vi "UI-电源头正面标签凹凸检测.vi"(8 "error in (no error)":errorcluster caption="错误输入（无错误）", 11 "名称或相对路径":string="Template Program") -> (0 "error in (no error) 2":errorcluster caption="错误输入（无错误）")   [LabVIEW 2017]
uses:
  Picture/SaveButtom.ctl
  Global System.vi
  <vilib>/Utility/xml.llb/Write to XML File(string).vi
panel:
  in  "获取图像":bool
  in  "创建模板":bool
  in  "保存图像":bool
  out "添加的路径":path
  in  "刷新":bool
  in  "测试按钮":bool
  in  "保存按钮":bool
  in  "Main":enum32{"主参数", "颜色模板匹配参数 ", "测试效果"}(tab)
  in  "UI电源线正面凹凸基础参数":T1={"IsNorImage"=TRUE, "Exposure Values"=100289, "ImagePath"=path "C:/Users/hedongpo/Desktop/514-hdp/Alignment Assemble System/Test Picture/B/3.bmp"} caption="参数界面" {"Exposure Values" scale=0.0..200000.0}
  in  "UI电源线正面凹凸参数":T2={"Min Radius"=7.0, "Max Radius"=11.0, "Max Number"=11.0}
  out "结果":bool
  out "原始图像":T3(plugin-control)
  out "大小":i32
  out "路径输出":path
  in  "Vision Paramter Save Buttom":T4
  out "system time":string
  in  "取消按钮":bool
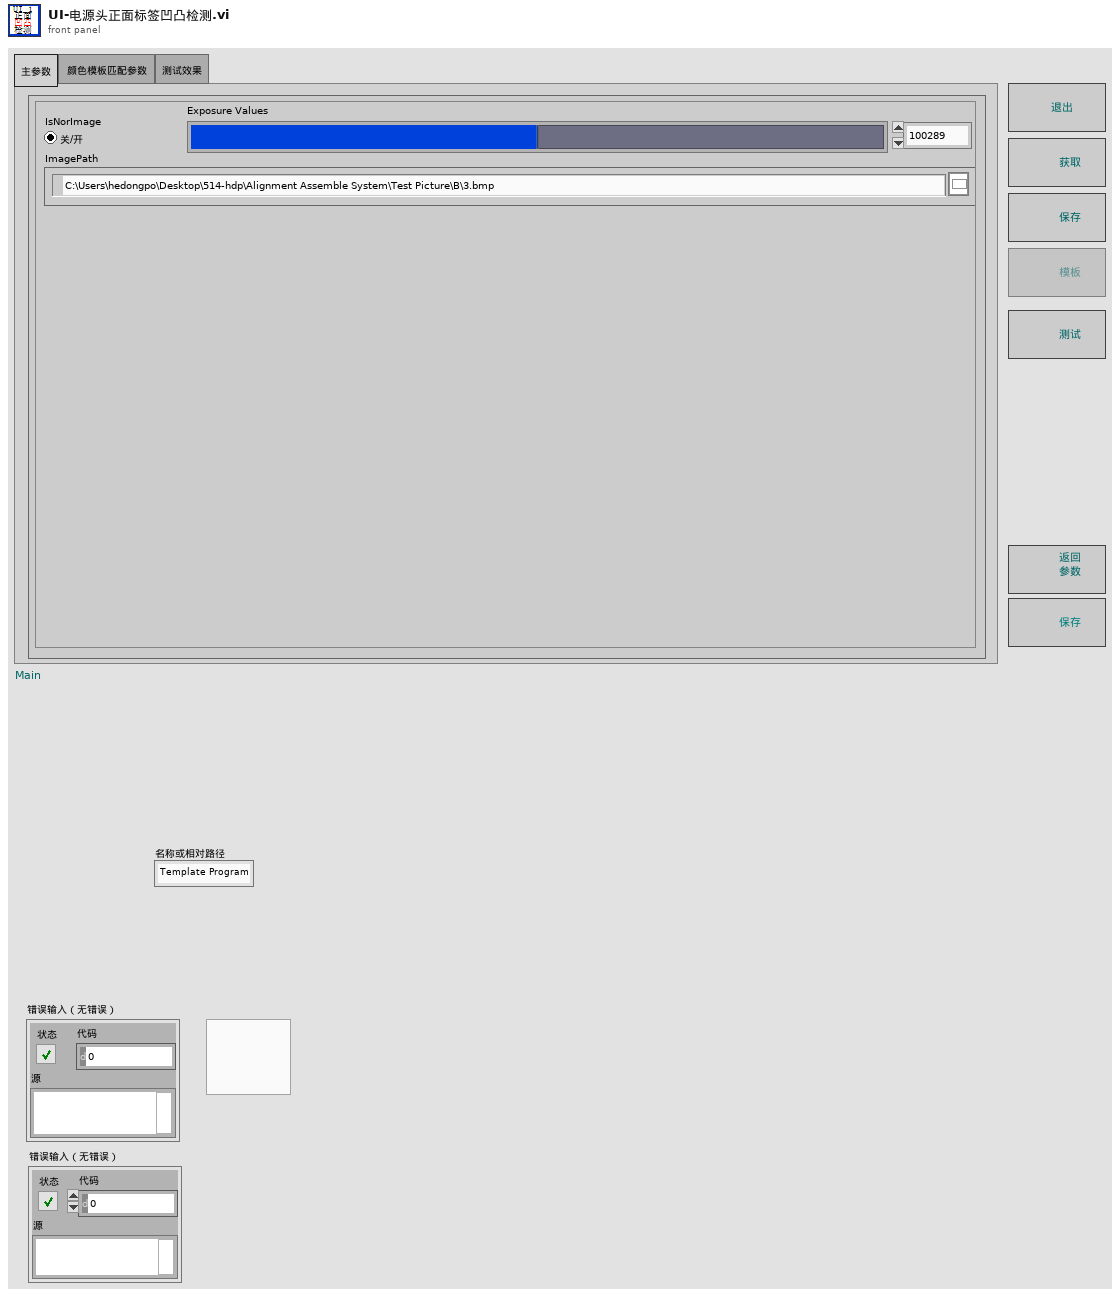
[diagram p1: front panel]
types:
  T1 = cluster{"IsNorImage":bool, "Exposure Values":u32, "ImagePath":path}
  T2 = cluster{"Min Radius":sgl, "Max Radius":sgl, "Max Number":sgl}
  T3 = typedef "IMAQ Image.ctl" = refnum<image>
  T4 = typedef "SaveButtom.ctl" = bool
  T5 = cluster{"index":i32, "this vi":refnum<vi>, "error out":errorcluster}
  T6 = cluster{"master data":string, "priority":u16, "secondary data":string[]}
  T7 = cluster{"case name":string[], "queue array":refnum<queue>[]}
  T8 = cluster{"Pos. X":i32, "Pos. Y":i32, "Radius":i32, "Core Area":i32}[]
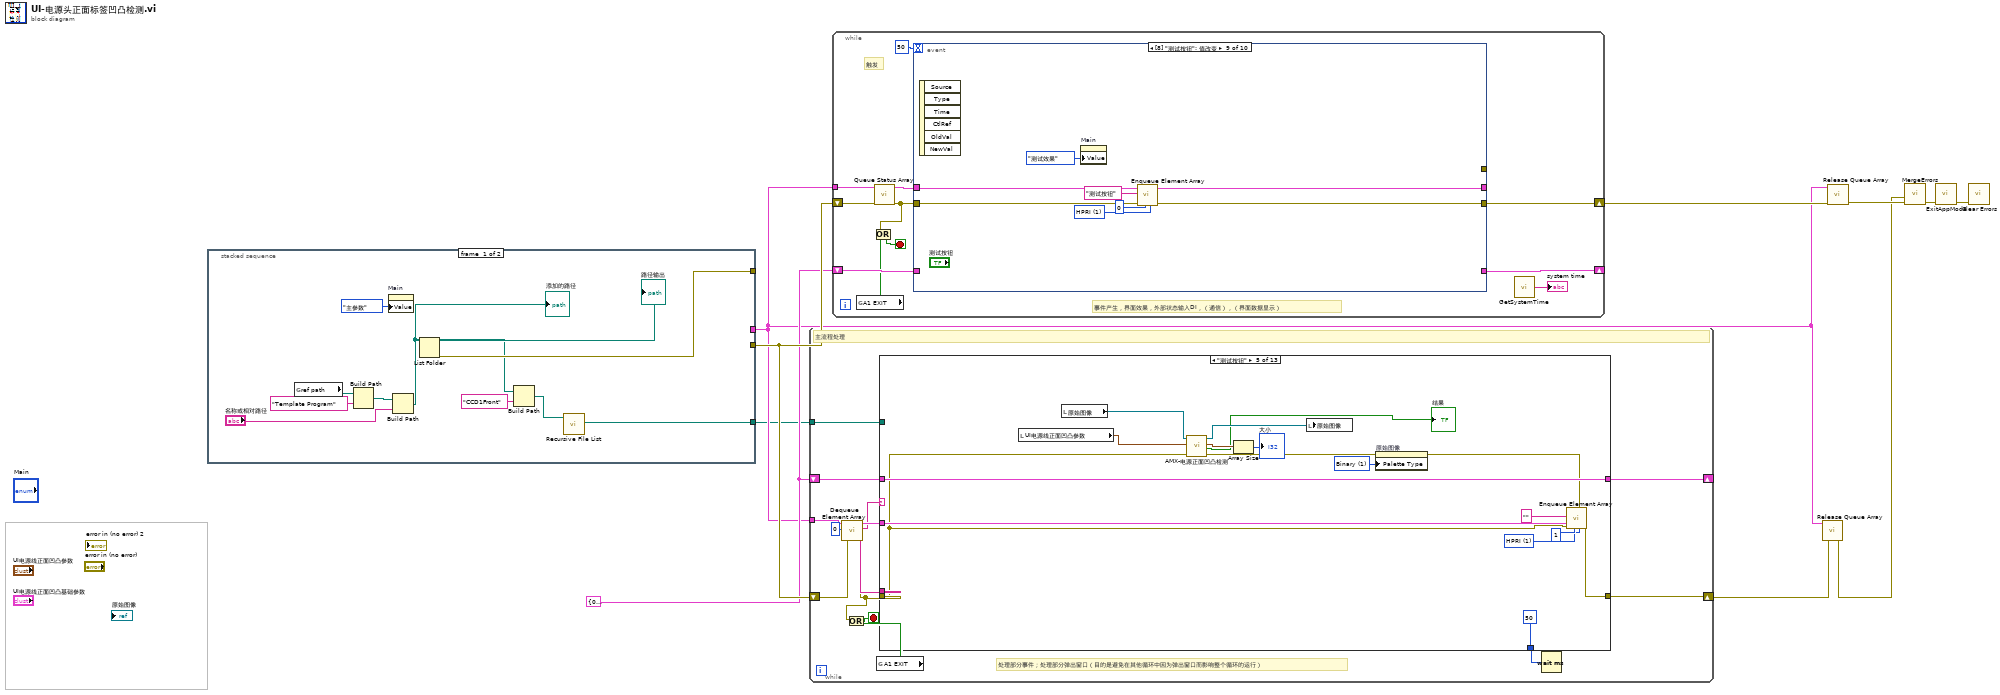
[diagram p0: block diagram]
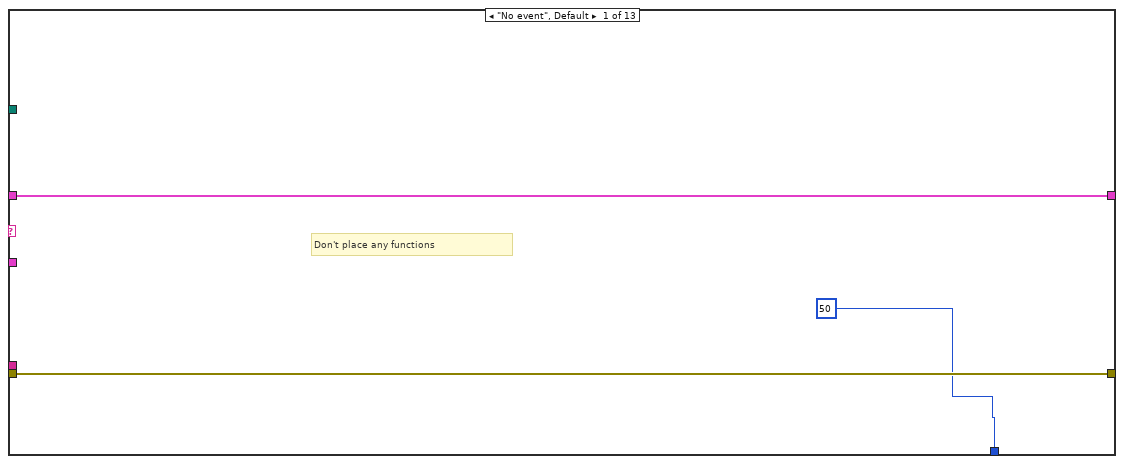
[diagram p2: hidden frame]
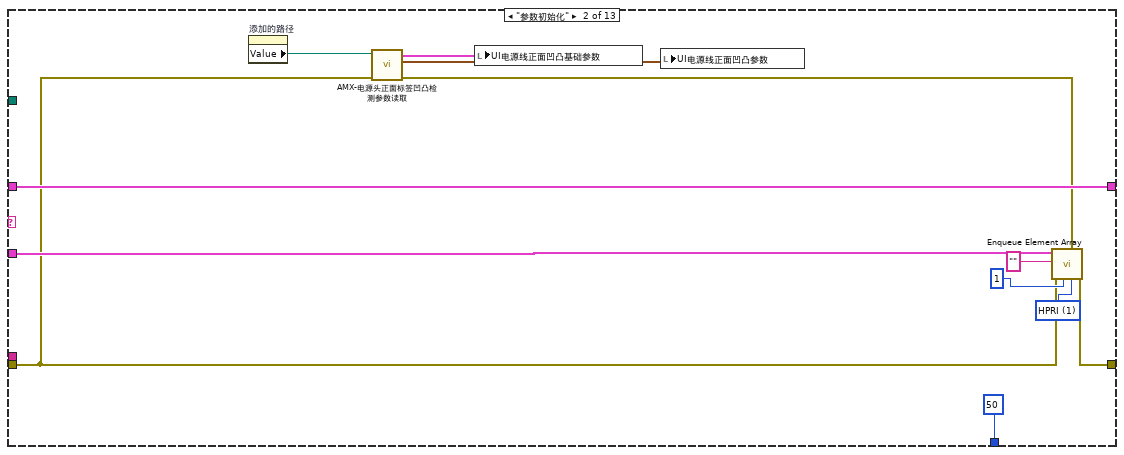
[diagram p3: hidden frame]
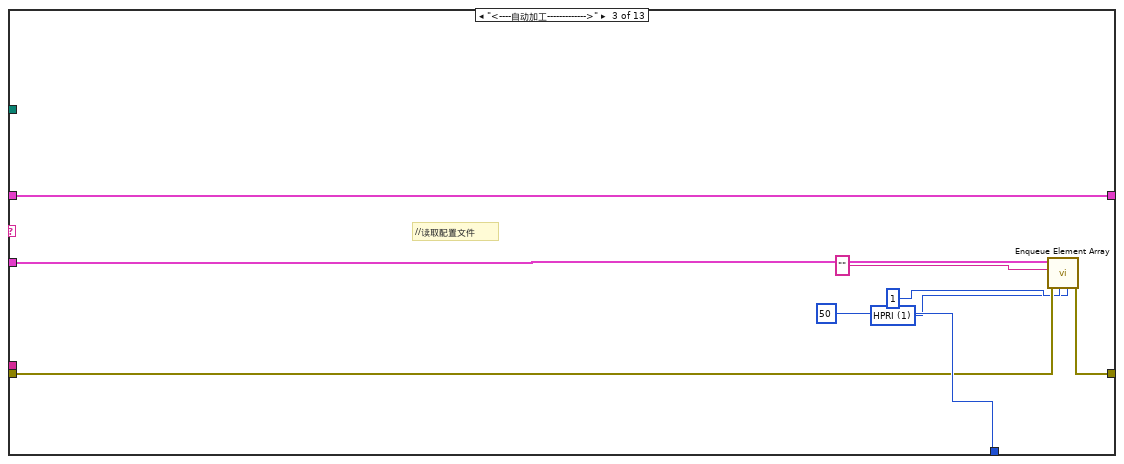
[diagram p4: hidden frame]
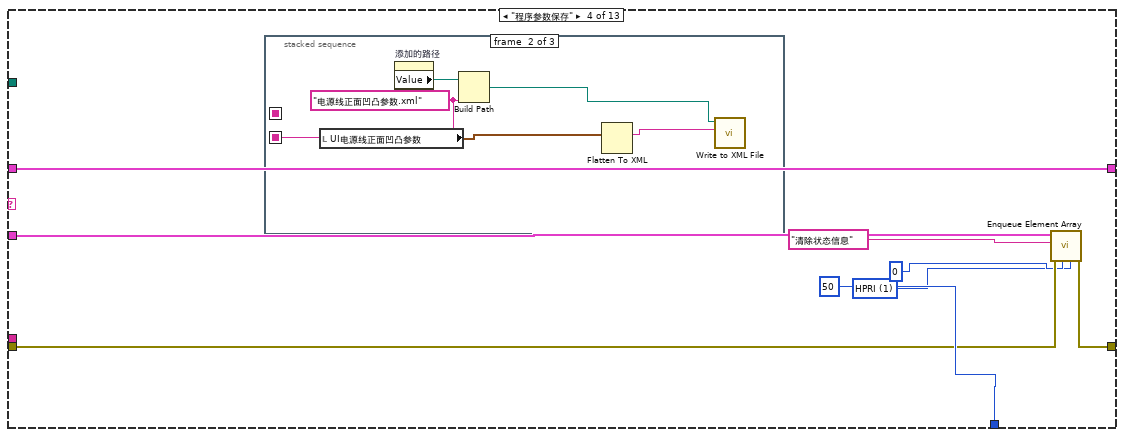
[diagram p5: hidden frame]
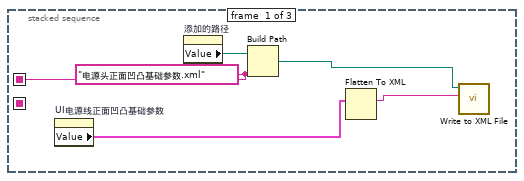
[diagram p6: hidden frame]
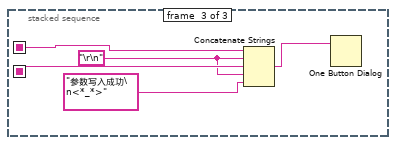
[diagram p7: hidden frame]
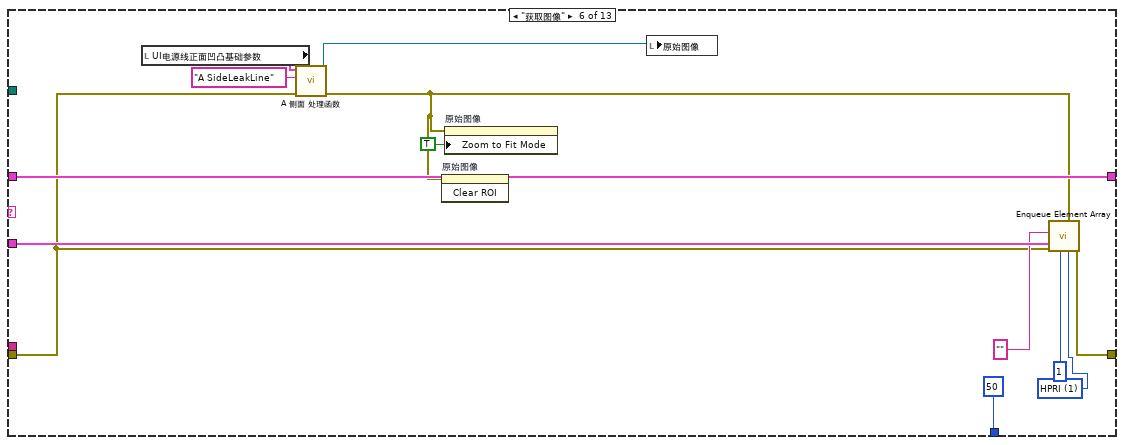
[diagram p8: hidden frame]
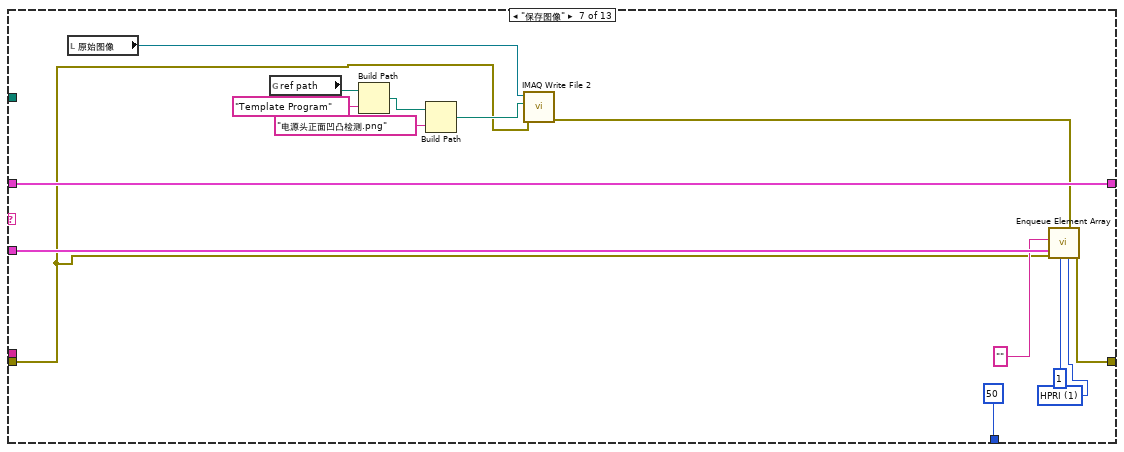
[diagram p9: hidden frame]
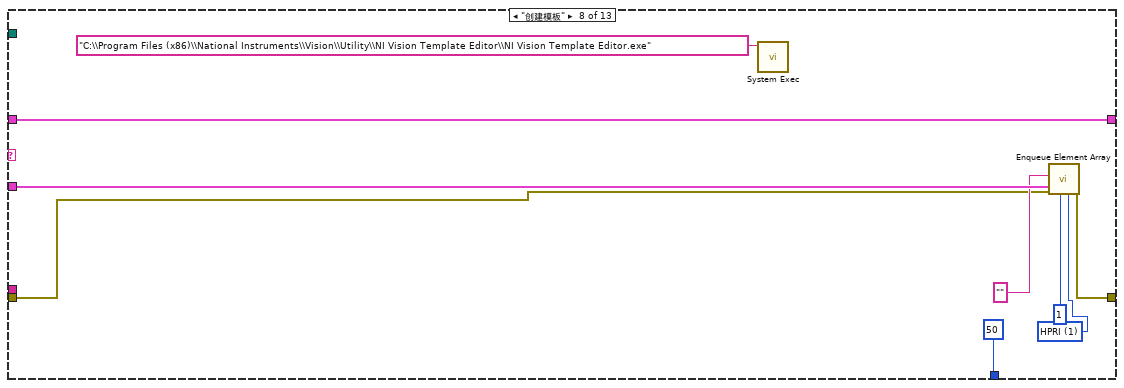
[diagram p10: hidden frame]
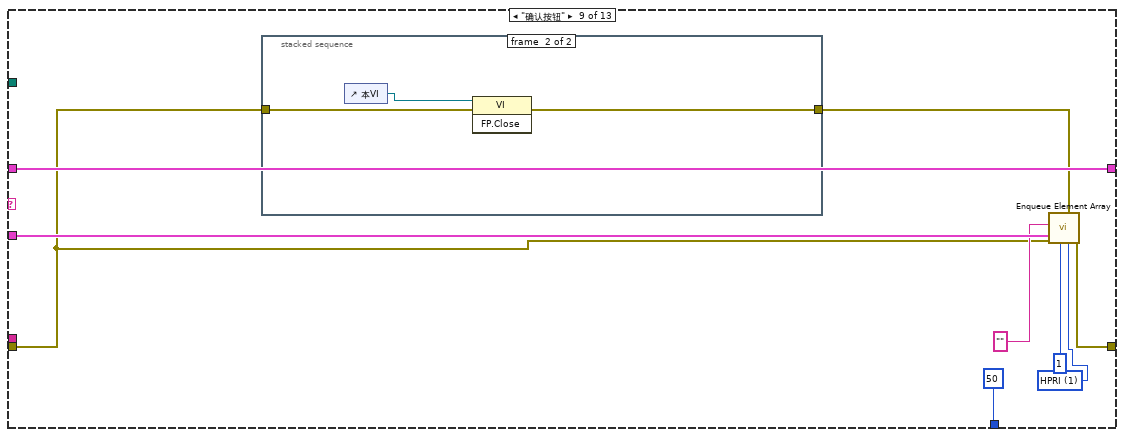
[diagram p11: hidden frame]
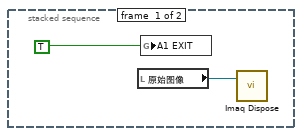
[diagram p12: hidden frame]
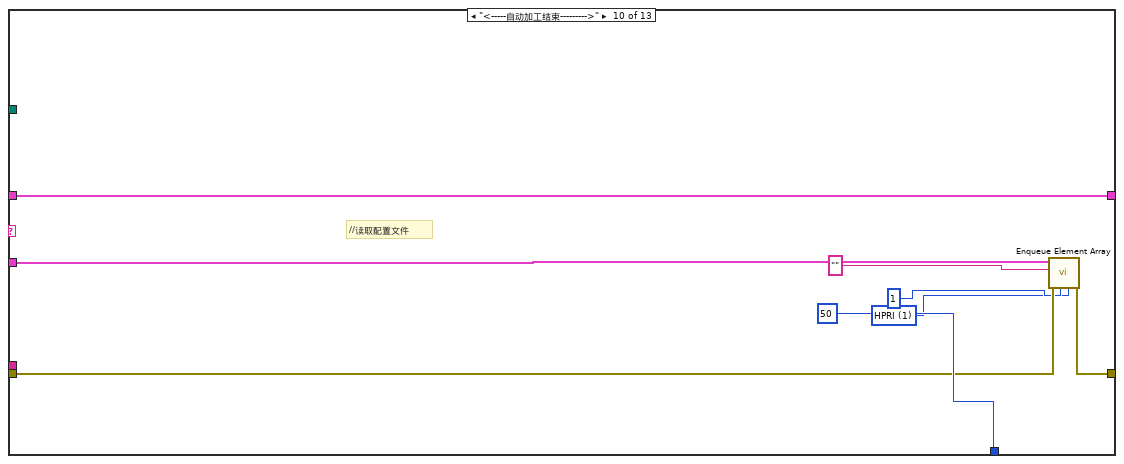
[diagram p13: hidden frame]
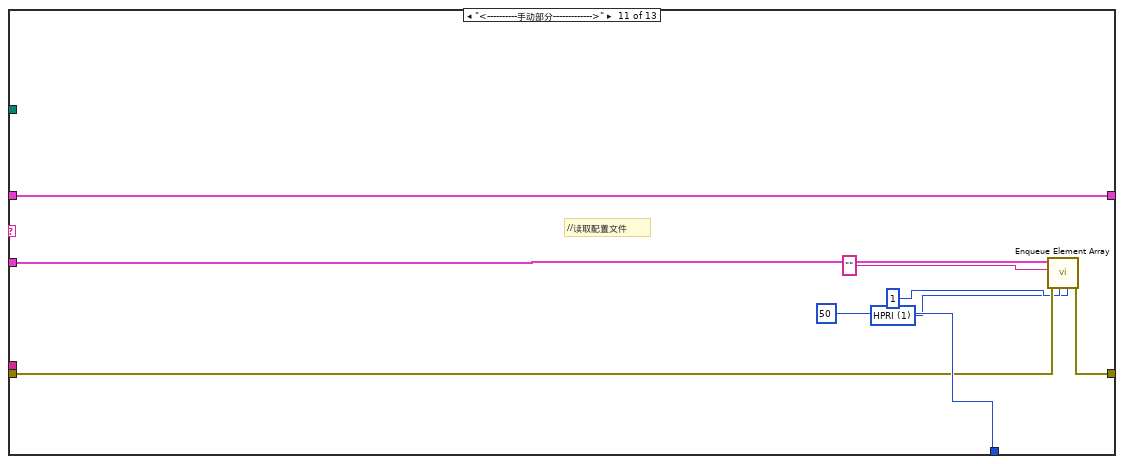
[diagram p14: hidden frame]
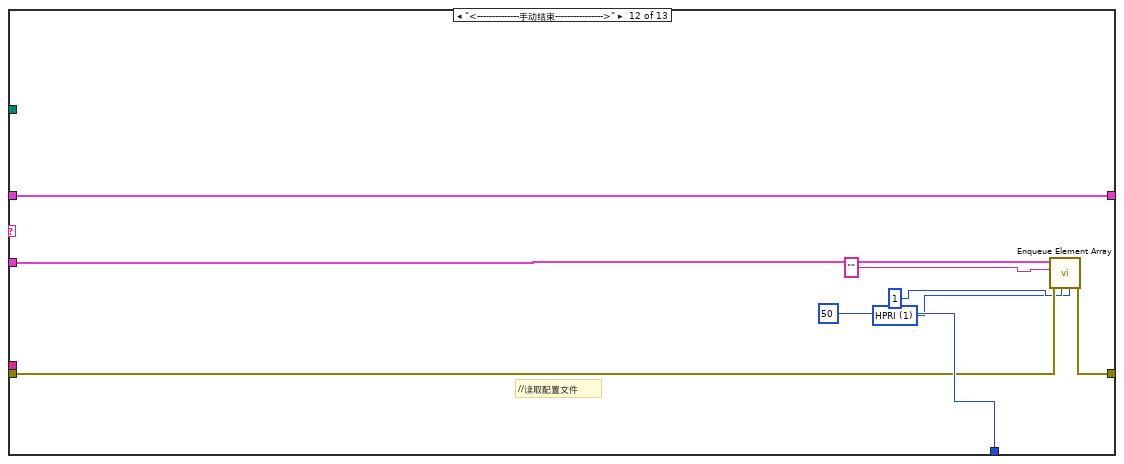
[diagram p15: hidden frame]
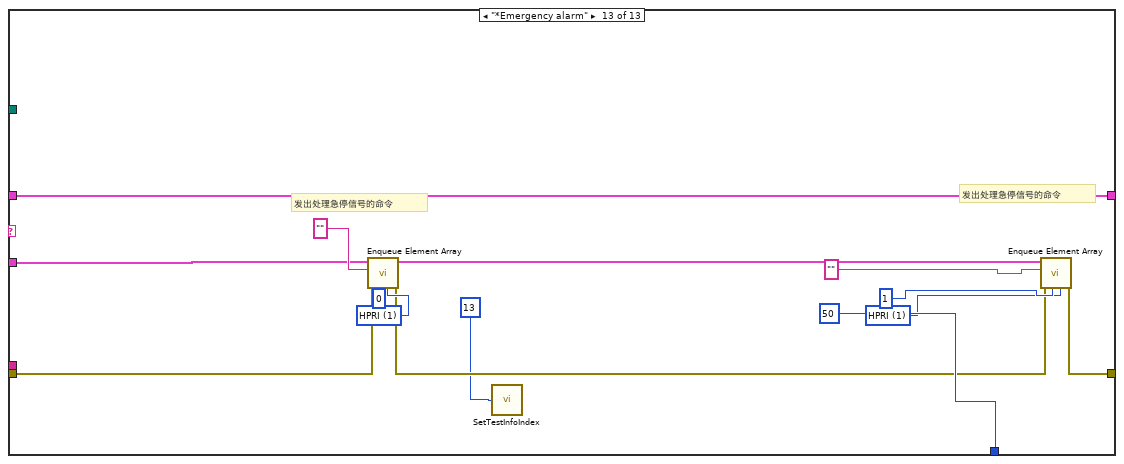
[diagram p16: hidden frame]
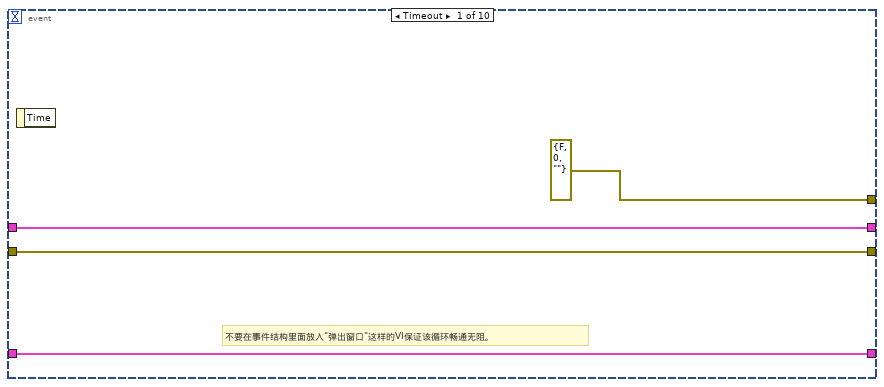
[diagram p17: hidden frame]
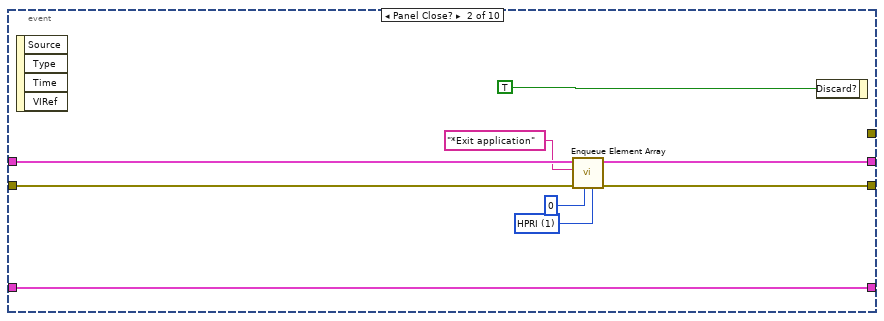
[diagram p18: hidden frame]
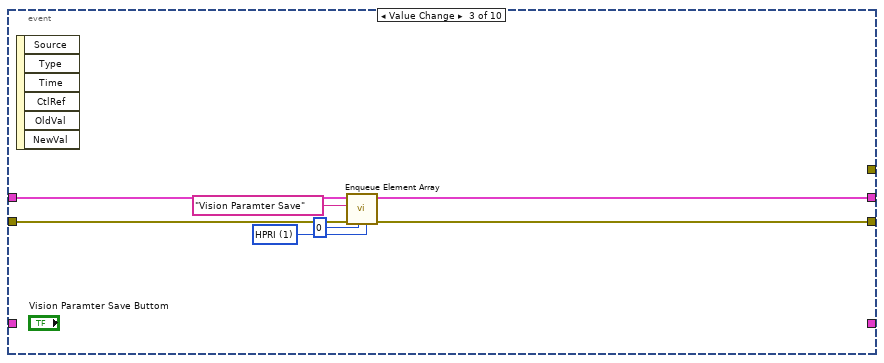
[diagram p19: hidden frame]
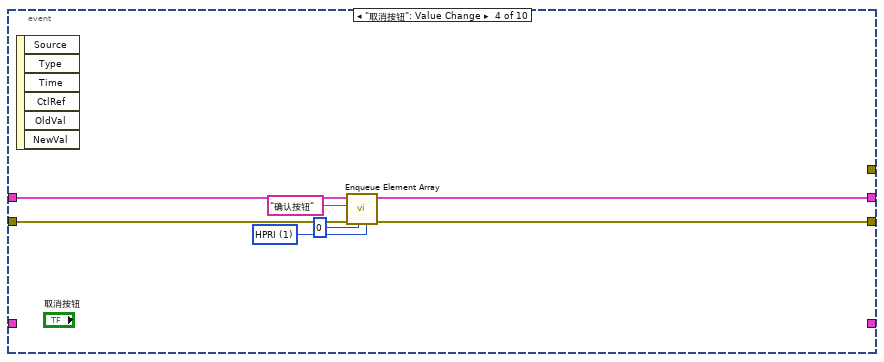
[diagram p20: hidden frame]
diagram:
  w5 = T5 {"index"=0, "this vi"=refnum, "error out"={"status"=FALSE, "code"=0, "source"=""}} ("parameter buffer")
  n1 = stacked-sequence {
    tunnel: [w20 _] -> _
    tunnel: [_ w23] -> w6
    tunnel: [_ w22] -> w2
    tunnel: [w11 _] -> w1
    frame #0 {
      n2 = global read "Global System.vi" "ref path"() -> (w18:path)
      n3 = Build Path(base path=w18, name or relative path="Template Program" ("名称或相对路径")) -> (appended path=w16:path)
      n4 = property on="Main" class="TabCtl (严格)"("Value"=enum32{"主参数", "颜色模板匹配参数 ", "测试效果"}."主参数" ("Main")) -> ()  [unwired: 2 in, 2 out]
      n5 = Build Path(base path=w16, name or relative path="名称或相对路径") -> (appended path=w12:path)
      "添加的路径" <- w12
      n6 = List Folder(path=w12) -> (path out=→"路径输出":path, error out=w20:errorcluster)  [unwired: 3 in, 2 out]
      n7 = Build Path(base path=w12, name or relative path="CCD1Front" ("名称或相对路径")) -> (appended path=w13:path)
      n8 = call <vilib>:"Recursive File List.vi"("Folder Path"=w13) -> ("All Files in Dir"=w11:path[])  [unwired: 6 in, 4 out]
    }
    frame #1 {
      w31 = string[] ["comm queue1", "data queue 11", "data queue 12", "data queue 13", "data queue 14"]  # queue name
      w32 = 4  # queue num
      w33 = T6 {"master data"="", "priority"=0, "secondary data"=[]}  # element data type
      n9 = call "Obtain Queue Array.vi"("queue name"=w31, "element data type"=w33, "queue num"=w32) -> ("error out"=w27:errorcluster, "queue out"=w28:T7)  [unwired: 2 in, 1 out]
      n10 = call "Enqueue Element Array.vi"("queue index"=0, "error in"=w27, "master data"="参数初始化", "queue in"=w28) -> ("error out"=w26:errorcluster, "queue out"=w25:T7)  [unwired: 6 in]
      n11 = disable-structure shown="启用" {
        disable-tunnel: w26 -> [w39 w40]
        disable-tunnel: w25 -> [w38 w41]
        disable-tunnel: "Loading Variable" ("master data") -> [w37 _]
        disable-tunnel: [w35 w40] -> w23
        disable-tunnel: [w34 w41] -> w22
        frame Disabled {
          n12 = call "Enqueue Element Array.vi"("queue index"=12, "error in"=w39, "master data"=w37, "queue in"=w38) -> ("error out"=w35:errorcluster, "queue out"=w34:T7)  [unwired: 6 in]
        }
        frame Enabled {
        }
      }
    }
  }
  n13 = while {
    shift-right: [w55] -> w4
    shift-left: w6 -> [w46]
    shift-right: [w52] -> _
    shift-left: w5 -> [w53]
    tunnel: w2 -> [w48]
    tunnel: w1 -> [w42]
    stop <- w43 stop-if-true
    # "处理部分事件；处理部分弹出窗口（目的是避免在其他循环中因为弹出窗口而影响整个循环的运行）"
    # "主流程处理"
    n14 = call "Dequeue Element Array.vi"("queue in"=w48, "queue index"=0, "error in"=w46) -> ("queue out"=w51:T7, "master data"=w50:string, "secondary data"=w49:string[], "error out"=w45:errorcluster)  [unwired: 2 in, 1 out]
    n15 = global read "Global System.vi" "A1 EXIT"() -> (w44:bool)
    n16 = Or(x=w45, y=w44) -> (x .or. y?=w43:bool)
    n17 = case shown="\"测试按钮\"" w50 {
      tunnel: w51 -> [_ w69 w77 w79 w117 w130 w145 w154 w163 w176 w184 w192 w198]
      tunnel: w45 -> [w57 w63 w73 w83 w109 w121 w132 w148 w157 w172 w180 w188 w195]
      tunnel: [w57 w68 w76 w85 w116 w129 w144 w153 w162 w175 w183 w191 w206] -> w55
      tunnel: [50 50 50 50 50 50 50 50 50 50 50 50 50] -> w54
      tunnel: w53 -> [w58 w64 w74 w80 w112 w125 w140 w149 w158 w173 w181 w189 w204]
      tunnel: [w58 w64 w74 w80 w112 w125 w140 w149 w158 w173 w181 w189 w204] -> w52
      tunnel: w49 -> [_ _ _ _ _ _ _ _ _ _ _ _ _]
      tunnel: w42 -> [_ _ _ _ _ _ _ _ _ _ _ _ _]
      frame "No event", Default {
        # "Don't place any functions"
      }
      frame "参数初始化" {
        w65 = u16 1 items=["HPRI"=1, "LPRI"=0] ("priority")
        n18 = property on="添加的路径" class="Path"() -> ("Value"=w61:path)  [unwired: 2 in, 2 out]
        n19 = call "AMX-电源头正面标签凹凸检测参数读取.vi"("error in (no error)"=w63, "基路径"=w61) -> ("error out"=w62:errorcluster, "UI电源线正面凹凸参数"=w59:T2, "UI电源线正面漏线基础参数"=w60:T1)  [unwired: 6 in]
        n20 = local write "UI电源线正面凹凸基础参数"(w60) -> ()
        n21 = local write "UI电源线正面凹凸参数"(w59) -> ()
        n22 = call "Enqueue Element Array.vi"("priority"=w65, "device error in"=w62, "queue index"=1, "error in"=w63, "master data"="" ("Element 1"), "queue in"=w69) -> ("error out"=w68:errorcluster)  [unwired: 4 in, 1 out]
      }
      frame "<----自动加工------------->" {
        w71 = u16 1 items=["HPRI"=1, "LPRI"=0] ("priority")
        # "//读取配置文件"
        n23 = call "Enqueue Element Array.vi"("priority"=w71, "queue index"=1, "error in"=w73, "master data"="" ("Element 1"), "queue in"=w77) -> ("error out"=w76:errorcluster)  [unwired: 5 in, 1 out]
      }
      frame "程序参数保存" {
        w81 = u16 1 items=["HPRI"=1, "LPRI"=0] ("priority")
        n24 = stacked-sequence {
          seq-local: [w87 _ _] -> [_ _ w100]
          seq-local: [_ w93 _] -> [_ _ w98]
          frame #0 {
            w87 = "电源头正面凹凸基础参数.xml" ("名称或相对路径")
            n25 = property on="UI电源线正面凹凸基础参数" class="Clust (严格)"() -> ("Value"=w90:T1)  [unwired: 2 in, 2 out]
            n26 = property on="添加的路径" class="Path"() -> ("Value"=w91:path)  [unwired: 2 in, 2 out]
            n27 = Build Path(base path=w91, name or relative path=w87) -> (appended path=w88:path)
            n28 = Flatten To XML(anything=w90) -> (xml string=w89:string)
            n29 = call-poly <vilib>:"Write to XML File.vi"("XML Input"=w89, "XML File Path"=w88) -> ()  [unwired: 7 in, 3 out]
          }
          frame #1 {
            w93 = "电源线正面凹凸参数.xml" ("名称或相对路径")
            n30 = local read "UI电源线正面凹凸参数"() -> (w92:T2)
            n31 = property on="添加的路径" class="Path"() -> ("Value"=w96:path)  [unwired: 2 in, 2 out]
            n32 = Build Path(base path=w96, name or relative path=w93) -> (appended path=w94:path)
            n33 = Flatten To XML(anything=w92) -> (xml string=w95:string)
            n34 = call-poly <vilib>:"Write to XML File.vi"("XML Input"=w95, "XML File Path"=w94) -> ()  [unwired: 7 in, 3 out]
          }
          frame #2 {
            w97 = "\r\n"
            n35 = Concatenate Strings(w100, w97, w98, w97, "参数写入成功\n<*_*>" ("消息")) -> (w99:string)
            n36 = One Button Dialog(message=w99) -> ()  [unwired: 1 in, 1 out]
          }
        }
        n37 = call "Enqueue Element Array.vi"("priority"=w81, "queue index"=0, "error in"=w83, "master data"="清除状态信息" ("Element 1"), "queue in"=w79) -> ("error out"=w85:errorcluster)  [unwired: 5 in, 1 out]
      }
      frame "测试按钮" {
        w104 = u32 1 items=["Grayscale", "Binary", "Gradient", "Rainbow", "Temperature", "User Defined", "Binary 16 Bit", "Gradient 16 Bit", "Rainbow 16 Bit", "Temperature 16 Bit", "User Defined 16 Bit"] ("Palette:Palette Type")
        w113 = u16 1 items=["HPRI"=1, "LPRI"=0] ("priority")
        n38 = local read "UI电源线正面凹凸参数"() -> (w103:T2)
        n39 = local read "原始图像"() -> (w111:T3)
        n40 = call "AMX-电源正面凹凸检测.vi"("error in (no error)"=w109, "UI电源线正面漏线参数"=w103, "Image in"=w111) -> ("error out"=w106:errorcluster, "x >= y?"=→"结果":bool, "Circles Data (calibrated) (Circle Detection 1)"=w108:T8, "Image out"=w110:T3)  [unwired: 5 in]
        n41 = Array Size(array=w108) -> (size(s)=→"大小":i32)
        n42 = local write "原始图像"(w110) -> ()
        n43 = property on="原始图像" class="ImageControl"(error in=w106, "Palette Type"=w104) -> (error out=w105:errorcluster)  [unwired: 1 in, 1 out]
        n44 = call "Enqueue Element Array.vi"("priority"=w113, "device error in"=w105, "queue index"=1, "error in"=w109, "master data"="" ("Element 1"), "queue in"=w117) -> ("error out"=w116:errorcluster)  [unwired: 4 in, 1 out]
      }
      frame "获取图像" {
        w126 = u16 1 items=["HPRI"=1, "LPRI"=0] ("priority")
        n45 = local read "UI电源线正面凹凸基础参数"() -> (w123:T1)
        n46 = call "A 侧面 处理函数.vi"("error in (no error)"=w121, "Image Name"="A SideLeakLine", "ParamsUI"=w123) -> ("error out"=w119:errorcluster, "Image out"=w122:T3)  [unwired: 5 in, 2 out]
        n47 = invoke on="原始图像" class="ImageControl" method="Clear ROI"(error in=w119) -> ()  [unwired: 2 in, 3 out]
        n48 = property on="原始图像" class="ImageControl"(error in=w119, "Zoom to Fit Mode"=TRUE) -> ()  [unwired: 1 in, 2 out]
        n49 = local write "原始图像"(w122) -> ()
        n50 = call "Enqueue Element Array.vi"("priority"=w126, "device error in"=w119, "queue index"=1, "error in"=w121, "master data"="" ("Element 1"), "queue in"=w130) -> ("error out"=w129:errorcluster)  [unwired: 4 in, 1 out]
      }
      frame "保存图像" {
        w141 = u16 1 items=["HPRI"=1, "LPRI"=0] ("priority")
        n51 = local read "原始图像"() -> (w133:T3)
        n52 = global read "Global System.vi" "ref path"() -> (w139:path)
        n53 = Build Path(base path=w139, name or relative path="Template Program" ("名称或相对路径")) -> (appended path=w137:path)
        n54 = Build Path(base path=w137, name or relative path="电源头正面凹凸检测.png" ("名称或相对路径")) -> (appended path=w135:path)
        n55 = call-poly "IMAQ Write File 2"("error in (no error)"=w132, "File Path"=w135, "Image"=w133) -> ("error out"=w134:errorcluster)  [unwired: 7 in, 1 out]
        n56 = call "Enqueue Element Array.vi"("priority"=w141, "device error in"=w134, "queue index"=1, "error in"=w132, "master data"="" ("Element 1"), "queue in"=w145) -> ("error out"=w144:errorcluster)  [unwired: 4 in, 1 out]
      }
      frame "创建模板" {
        w150 = u16 1 items=["HPRI"=1, "LPRI"=0] ("priority")
        n57 = call <vilib>:"System Exec.vi"("command line"="C:\\Program Files (x86)\\National Instruments\\Vision\\Utility\\NI Vision Template Editor\\NI Vision Template Editor.exe") -> ()  [unwired: 7 in, 4 out]
        n58 = call "Enqueue Element Array.vi"("priority"=w150, "queue index"=1, "error in"=w148, "master data"="" ("Element 1"), "queue in"=w154) -> ("error out"=w153:errorcluster)  [unwired: 5 in, 1 out]
      }
      frame "确认按钮" {
        w159 = u16 1 items=["HPRI"=1, "LPRI"=0] ("priority")
        n59 = stacked-sequence {
          tunnel: w157 -> [_ w168]
          tunnel: [_ w167] -> w156
          frame #0 {
            n60 = local read "原始图像"() -> (w165:T3)
            n61 = global write "Global System.vi" "A1 EXIT"(TRUE ("EXIT")) -> ()
            n62 = call "Imaq Dispose"("Image"=w165) -> ()  [unwired: 5 in, 1 out]
          }
          frame #1 {
            n63 = control-ref of="本VI"() -> (w169:refnum<vi>)
            n64 = invoke class="VI" method="FP.Close"(reference=w169, error in=w168) -> (error out=w167:errorcluster)  [unwired: 1 in, 2 out]
          }
        }
        n65 = call "Enqueue Element Array.vi"("priority"=w159, "device error in"=w156, "queue index"=1, "error in"=w157, "master data"="" ("Element 1"), "queue in"=w163) -> ("error out"=w162:errorcluster)  [unwired: 4 in, 1 out]
      }
      frame "<-----自动加工结束--------->" {
        w170 = u16 1 items=["HPRI"=1, "LPRI"=0] ("priority")
        # "//读取配置文件"
        n66 = call "Enqueue Element Array.vi"("priority"=w170, "queue index"=1, "error in"=w172, "master data"="" ("Element 1"), "queue in"=w176) -> ("error out"=w175:errorcluster)  [unwired: 5 in, 1 out]
      }
      frame "<----------手动部分------------->" {
        w178 = u16 1 items=["HPRI"=1, "LPRI"=0] ("priority")
        # "//读取配置文件"
        n67 = call "Enqueue Element Array.vi"("priority"=w178, "queue index"=1, "error in"=w180, "master data"="" ("Element 1"), "queue in"=w184) -> ("error out"=w183:errorcluster)  [unwired: 5 in, 1 out]
      }
      frame "<--------------手动结束---------------->" {
        w186 = u16 1 items=["HPRI"=1, "LPRI"=0] ("priority")
        # "//读取配置文件"
        n68 = call "Enqueue Element Array.vi"("priority"=w186, "queue index"=1, "error in"=w188, "master data"="" ("Element 1"), "queue in"=w192) -> ("error out"=w191:errorcluster)  [unwired: 5 in, 1 out]
      }
      frame "*Emergency alarm" {
        w201 = u16 1 items=["HPRI"=1, "LPRI"=0] ("priority")
        w202 = u16 1 items=["HPRI"=1, "LPRI"=0] ("priority")
        # "发出处理急停信号的命令"
        # "发出处理急停信号的命令"
        n69 = call "Enqueue Element Array.vi"("priority"=w201, "queue index"=0, "error in"=w195, "master data"="" ("Element 1"), "queue in"=w198) -> ("error out"=w196:errorcluster, "queue out"=w197:T7)  [unwired: 5 in]
        n70 = call "SetTestInfoIndex.vi"("test info index"=13) -> ()
        n71 = call "Enqueue Element Array.vi"("priority"=w202, "queue index"=1, "error in"=w196, "master data"="" ("Element 1"), "queue in"=w197) -> ("error out"=w206:errorcluster)  [unwired: 5 in, 1 out]
      }
    }
    n72 = Wait (ms)(milliseconds to wait=w54) -> ()  [unwired: 1 out]
  }
  n73 = while {
    shift-right: [w211] -> w7
    shift-left: w6 -> [w215]
    shift-right: [w213] -> _
    shift-left: w5 -> [w214]
    tunnel: w2 -> [w217]
    stop <- w208 stop-if-true
    # "触发"
    # "事件产生，界面效果，外部状态输入DI，（通信），（界面数据显示）"
    n74 = global read "Global System.vi" "A1 EXIT"() -> (w209:bool)
    n75 = call "Queue Status Array.vi"("error in (no error)"=w215, "queue in"=w217) -> ("error out"=w210:errorcluster, "queue out"=w212:T7)  [unwired: 4 in]
    n76 = Or(x=w210, y=w209) -> (x .or. y?=w208:bool)
    n77 = event shown="[8] \"测试按钮\": 值改变" {
      selector: _ -> [_ _ _ _ _ _ _ _ _ _]
      dyn-events: _ -> [_ _ _ _ _ _ _ _ _ _]
      timeout: 50 -> [_ _ _ _ _ _ _ _ _ _]
      tunnel: w214 -> [w222 w230 _ _ _ _ _ _ _ _]
      tunnel: [w222 w230 _ _ _ _ _ _ _ _] -> w213
      tunnel: [errorcluster {"status"=FALSE, "code"=0, "source"=""} ("error out") _ _ _ _ _ _ _ _ _] -> _
      tunnel: w212 -> [w220 w229 w235 w242 w249 w257 w264 w271 w279 w287]
      tunnel: w210 -> [w219 w228 w234 w241 w248 w256 w263 w270 w278 w286]
      tunnel: [w219 w227 w232 w239 w246 w254 w261 w268 w276 w284] -> w211
      tunnel: [w220 w226 w233 w240 w247 w255 w262 w269 w277 w285] -> _
      event Timeout {
        # "不要在事件结构里面放入\"弹出窗口\"这样的VI保证该循环畅通无阻。"
        n78 = event-data() -> ()  [unwired: 1 in, 1 out]
      }
      event Panel Close? {
        w224 = u16 1 items=["HPRI"=1, "LPRI"=0] ("priority")
        n79 = event-data() -> ()  [unwired: 1 in, 4 out]
        n80 = call "Enqueue Element Array.vi"("priority"=w224, "queue index"=0, "error in"=w228, "master data"="*Exit application", "queue in"=w229) -> ("error out"=w227:errorcluster, "queue out"=w226:T7)  [unwired: 5 in]
        n81 = event-data("Discard?"=TRUE) -> ()  [unwired: 1 in, 1 out]
      }
      event Value Change {
        w237 = u16 1 items=["HPRI"=1, "LPRI"=0] ("priority")
        n82 = event-data() -> ()  [unwired: 1 in, 6 out]
        n83 = call "Enqueue Element Array.vi"("priority"=w237, "queue index"=0, "error in"=w234, "master data"="Vision Paramter Save", "queue in"=w235) -> ("error out"=w232:errorcluster, "queue out"=w233:T7)  [unwired: 5 in]
      }
      event "取消按钮": Value Change {
        w244 = u16 1 items=["HPRI"=1, "LPRI"=0] ("priority")
        n84 = event-data() -> ()  [unwired: 1 in, 6 out]
        n85 = call "Enqueue Element Array.vi"("priority"=w244, "queue index"=0, "error in"=w241, "master data"="确认按钮", "queue in"=w242) -> ("error out"=w239:errorcluster, "queue out"=w240:T7)  [unwired: 5 in]
      }
      event "保存按钮": Value Change {
        w251 = u16 1 items=["HPRI"=1, "LPRI"=0] ("priority")
        n86 = event-data() -> ()  [unwired: 1 in, 6 out]
        n87 = call "Enqueue Element Array.vi"("priority"=w251, "queue index"=0, "error in"=w248, "master data"="程序参数保存", "queue in"=w249) -> ("error out"=w246:errorcluster, "queue out"=w247:T7)  [unwired: 5 in]
      }
      event "获取图像": Value Change {
        w259 = u16 1 items=["HPRI"=1, "LPRI"=0] ("priority")
        n88 = event-data() -> ()  [unwired: 1 in, 6 out]
        n89 = property on="Main" class="TabCtl (严格)"("Value"=enum32{"主参数", "颜色模板匹配参数 ", "测试效果"}."测试效果" ("Main")) -> ()  [unwired: 2 in, 2 out]
        n90 = call "Enqueue Element Array.vi"("priority"=w259, "queue index"=0, "error in"=w256, "master data"="获取图像", "queue in"=w257) -> ("error out"=w254:errorcluster, "queue out"=w255:T7)  [unwired: 5 in]
      }
      event "保存图像": Value Change {
        w266 = u16 1 items=["HPRI"=1, "LPRI"=0] ("priority")
        n91 = event-data() -> ()  [unwired: 1 in, 6 out]
        n92 = call "Enqueue Element Array.vi"("priority"=w266, "queue index"=0, "error in"=w263, "master data"="保存图像", "queue in"=w264) -> ("error out"=w261:errorcluster, "queue out"=w262:T7)  [unwired: 5 in]
      }
      event "创建模板": Value Change {
        w273 = u16 1 items=["HPRI"=1, "LPRI"=0] ("priority")
        n93 = event-data() -> ()  [unwired: 1 in, 6 out]
        n94 = call "Enqueue Element Array.vi"("priority"=w273, "queue index"=0, "error in"=w270, "master data"="创建模板", "queue in"=w271) -> ("error out"=w268:errorcluster, "queue out"=w269:T7)  [unwired: 5 in]
      }
      event "测试按钮": Value Change {
        w281 = u16 1 items=["HPRI"=1, "LPRI"=0] ("priority")
        n95 = event-data() -> ()  [unwired: 1 in, 6 out]
        n96 = property on="Main" class="TabCtl (严格)"("Value"=enum32{"主参数", "颜色模板匹配参数 ", "测试效果"}."测试效果" ("Main")) -> ()  [unwired: 2 in, 2 out]
        n97 = call "Enqueue Element Array.vi"("priority"=w281, "queue index"=0, "error in"=w278, "master data"="测试按钮", "queue in"=w279) -> ("error out"=w276:errorcluster, "queue out"=w277:T7)  [unwired: 5 in]
      }
      event "刷新": Value Change {
        n98 = event-data() -> ()  [unwired: 1 in, 6 out]
        n99 = disable-structure shown="禁用" {
          disable-tunnel: w287 -> [w291 _]
          disable-tunnel: w286 -> [w290 _]
          disable-tunnel: [w289 _] -> w285
          disable-tunnel: [w288 _] -> w284
          frame Disabled {
            w293 = u16 1 items=["HPRI"=1, "LPRI"=0] ("priority")
            # "刷新"
            n100 = call "Enqueue Element Array.vi"("priority"=w293, "queue index"=0, "error in"=w290, "master data"="刷新", "queue in"=w291) -> ("error out"=w288:errorcluster, "queue out"=w289:T7)  [unwired: 5 in]
          }
          frame Enabled {
          }
        }
        n101 = property on="Main" class="TabCtl (严格)"("Value"=enum32{"主参数", "颜色模板匹配参数 ", "测试效果"}."颜色模板匹配参数 " ("Main")) -> ()  [unwired: 2 in, 2 out]
      }
    }
    n102 = call "GetSystemTime.vi"() -> ("date/time string"=→"system time":string)  [unwired: 7 in]
  }
  n103 = call "Release Queue Array.vi"("error in"=w4, "queue in"=w2) -> ("error out"=w3:errorcluster)  [unwired: 2 in, 3 out]
  n104 = call "Release Queue Array.vi"("error in"=w7, "queue in"=w2) -> ("error out"=w10:errorcluster)  [unwired: 2 in, 3 out]
  n105 = call "MergeErrors.vi"("error in 3 (no error)"=w3, "error in 4 (no error)"=w10) -> ("error out"=w9:errorcluster)  [unwired: 6 in]
  n106 = call "ExitAppMode.vi"("error in (no error)"=w9) -> ("error out"=w8:errorcluster)  [unwired: 10 in]
  n107 = call <vilib>:"Clear Errors.vi"("error in (no error)"=w8) -> ()  [unwired: 5 in, 2 out]
